vi "Final_Project_Intensity_Measurement.vi"() -> ()   [LabVIEW 2023]
doc: "This example shows how to get high accuracy DC voltage measurement."
uses:
  <instrlib>/Keithley DMM6500 DAQ6500 Series/Public/Data/Read (Single Point).vi
  <instrlib>/Keithley DMM6500 DAQ6500 Series/Keithley DMM6500 DAQ6500 Series.lvlib
panel:
  out "Intensity (W/m^2)":dbl
  out "Waveform Chart":dbl(graph)
  in  "stop":bool
  in  "Enable Average Filter (F: Disable)":bool
  in  "Input Impedance (0: 10Mohm)":i32(ring) items=["10Mohm", "Auto"]
  in  "Auto Zero (0: Enable)":u32(ring) items=["Enable", "Disable", "Once"]
  in  "Auto Range (T: Enable)":bool=TRUE
  in  "Average Filter Type (0: Repeat)":i32(ring) items=["Repeat", "Moving"]
  in  "Power Line Cycle (1)":dbl=10.0
  out "Voltage (V)":dbl
  in  "Average Count (10)":u32=10
  in  "Manual Range (0)":dbl=10.0
  in  "Channel List (\"101\")":string="101"
  in  "VISA resource name":refnum<visa-resource-name>
  # "(c) 2018-2022 National Instruments.  ALL RIGHTS RESERVED."
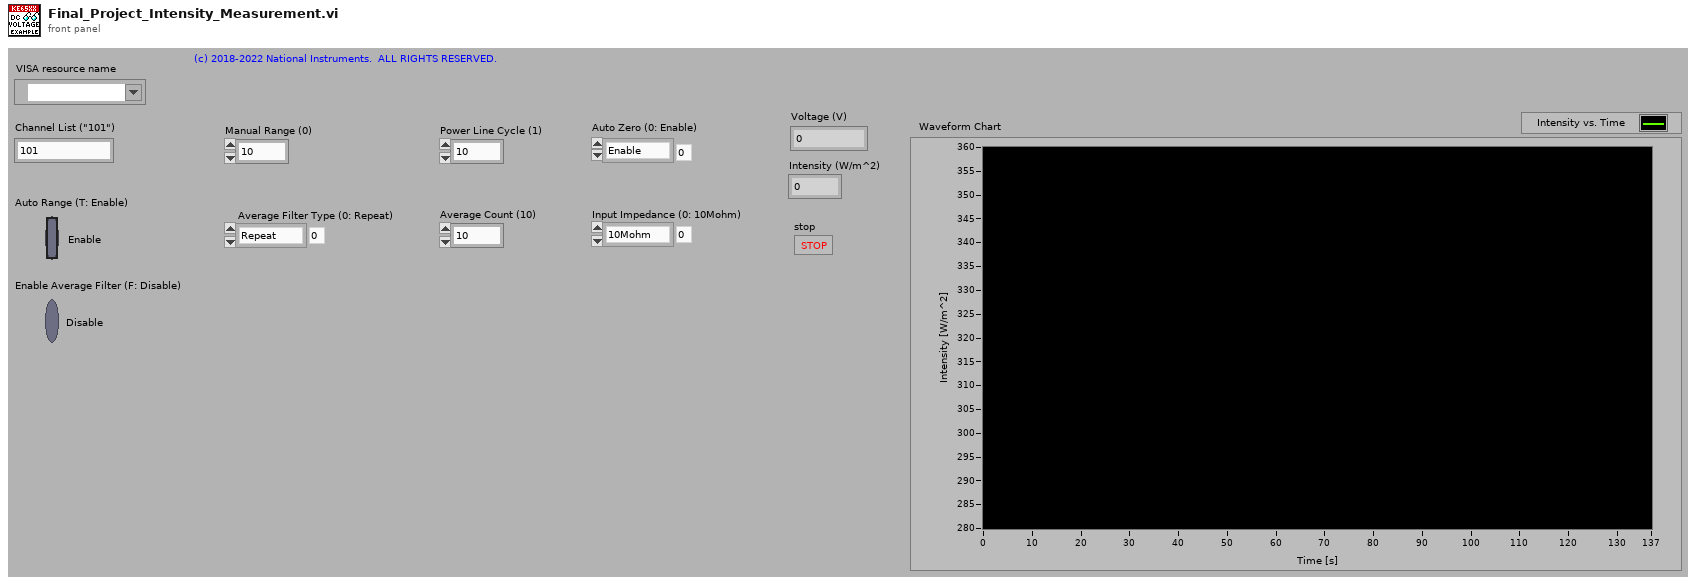
[diagram p1: front panel]
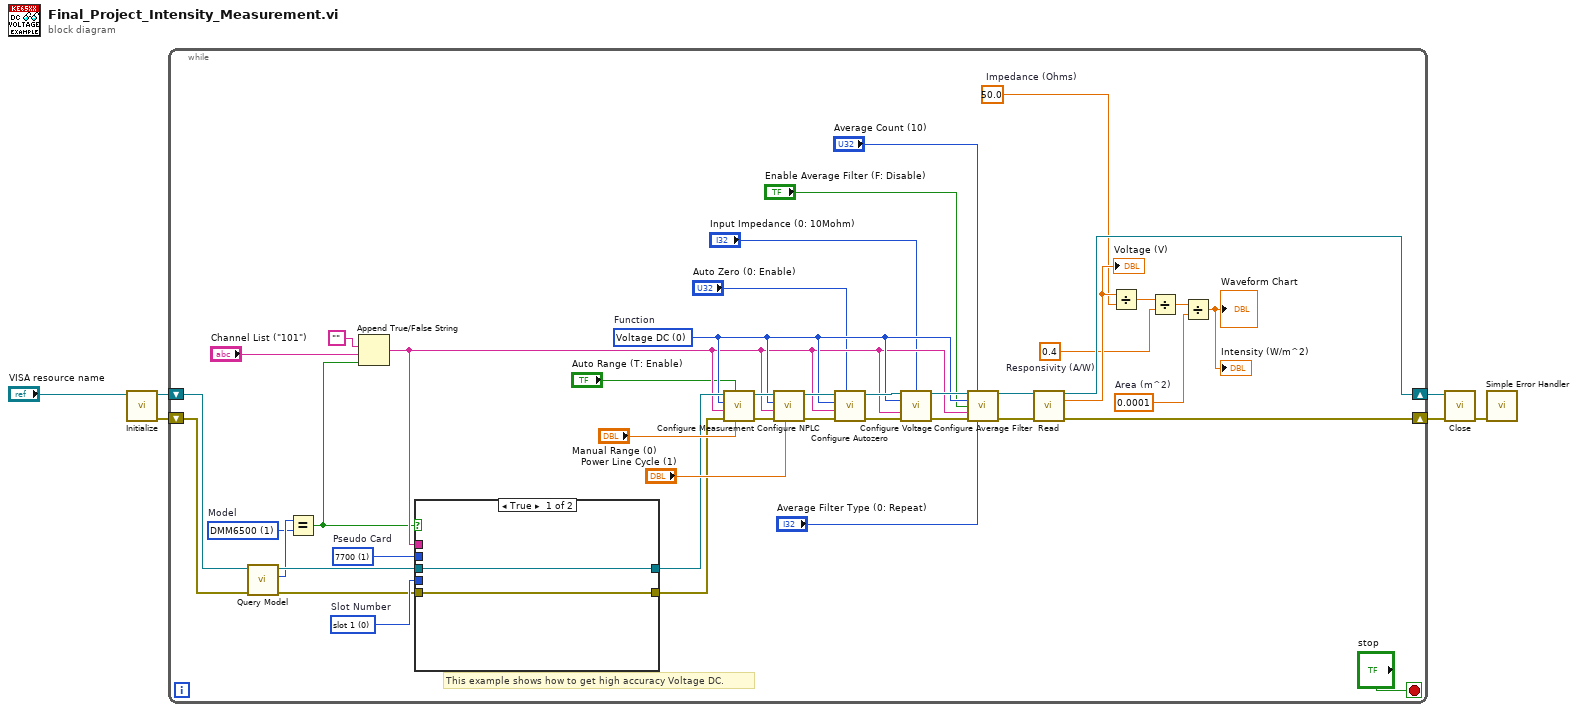
[diagram p0: block diagram]
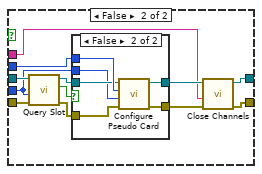
[diagram p2: hidden frame]
diagram:
  n1 = call <instrlib>:"Initialize.vi"("VISA resource name"="VISA resource name") -> ("error out"=w1:errorcluster, "VISA resource name out"=w2:refnum<visa-resource-name>)  [unwired: 9 in]
  n2 = while {
    shift-right: [w36] -> w3
    shift-left: w2 -> [w30]
    shift-right: [w37] -> w4
    shift-left: w1 -> [w28]
    stop <- "stop" stop-if-true
    w10 = 0.0001  # Area (m^2)
    w11 = 0.4  # Responsivity (A/W)
    w12 = 50.0  # Impedance (Ohms)
    w48 = 0 items=["slot 1", "slot 2"]  # Slot Number
    w49 = 1 items=["0", "7700", "7701", "7702", "7703", "7705", "7706", "7707", "7708", "7709", "7710", "7711", "7712"]  # Pseudo Card
    w24 = 0 items=[" Voltage DC", "Voltage AC", "Current DC", "Current AC", "Resistance", "4-wire Resistance", "Diode", "Capacitance", "Temperature", "Continuity", "Frequency", "Period", "Voltage Ratio", "Digitize Voltage", "Digitize Current"]  # Function
    w25 = 1 items=["", "DMM6500", "DAQ6510"]  # Model
    # "This example shows how to get high accuracy Voltage DC."
    n3 = call <instrlib>:"Query Model.vi"("error in (no error)"=w28, "VISA resource name"=w30) -> ("error out"=w27:errorcluster, "Model"=w26:i32, "VISA resource name out"=w29:refnum<visa-resource-name>)  [unwired: 7 in]
    n4 = Equal?(x=w26, y=w25) -> (x = y?=w20:bool)
    n5 = Append True/False String(1:w20, 2:"Channel List (\"101\")", 3:"") -> (0:w23:string)  [unwired: 1 in]
    n6 = case shown="True" w20 {
      tunnel: w49 -> [_ w63]
      tunnel: w48 -> [_ w53]
      tunnel: w29 -> [w51 w62]
      tunnel: w27 -> [w50 w55]
      tunnel: [w51 w60] -> w34
      tunnel: [w50 w58] -> w32
      tunnel: w23 -> [_ w57]
      frame True {
      }
      frame False {
        n7 = call <instrlib>:"Query Slot.vi"("error in (no error)"=w55, "Slot Number(0: slot 1)"=w53, "VISA resource name"=w62) -> ("error out"=w54:errorcluster, "Real Card In Slot"=w52:bool, "VISA resource name out"=w56:refnum<visa-resource-name>)  [unwired: 6 in]
        n8 = case shown="False" w52 {
          tunnel: w63 -> [_ w71]
          tunnel: [w65 w70] -> w61
          tunnel: [w64 w69] -> w59
          tunnel: w56 -> [w65 w68]
          tunnel: w54 -> [w64 w67]
          tunnel: w53 -> [_ w66]
          frame True {
          }
          frame False {
            n9 = call <instrlib>:"Configure Pseudo Card.vi"("error in (no error)"=w67, "Slot Number (0: slot1)"=w66, "Pseudo Card (0:No pseudocard)"=w71, "VISA resource name"=w68) -> ("error out"=w69:errorcluster, "VISA resource name out"=w70:refnum<visa-resource-name>)  [unwired: 6 in]
          }
        }
        n10 = call <instrlib>:"Close Channels.vi"("error in (no error)"=w59, "Channel List(\"\")"=w57, "VISA resource name"=w61) -> ("error out"=w58:errorcluster, "VISA resource name out"=w60:refnum<visa-resource-name>)  [unwired: 7 in]
      }
    }
    n11 = call <instrlib>:"Configure Measurement.vi"("Manual Range (1)"="Manual Range (0)", "Auto Range (T: Enable)"="Auto Range (T: Enable)", "error in (no error)"=w32, "Channel List(\"\")"=w23, "Function (0: Voltage DC)"=w24, "VISA resource name"=w34) -> ("error out"=w31:errorcluster, "VISA resource name out"=w33:refnum<visa-resource-name>)  [unwired: 4 in]
    n12 = call <instrlib>:"Configure NPLC.vi"("Power Line Cycle (1)"="Power Line Cycle (1)", "error in (no error)"=w31, "Channel List(\"\")"=w23, "Function (0: Voltage DC)"=w24, "VISA resource name"=w33) -> ("error out"=w45:errorcluster, "VISA resource name out"=w46:refnum<visa-resource-name>)  [unwired: 5 in]
    n13 = call <instrlib>:"Configure Autozero.vi"("Auto Zero (0: Enable)"="Auto Zero (0: Enable)", "error in (no error)"=w45, "Channel List(\"\")"=w23, "Function (0: Voltage DC)"=w24, "VISA resource name"=w46) -> ("error out"=w43:errorcluster, "VISA resource name out"=w44:refnum<visa-resource-name>)  [unwired: 5 in]
    n14 = call <instrlib>:"Configure Voltage.vi"("VISA resource name"=w44, "Input Impedance (0: 10Mohm)"="Input Impedance (0: 10Mohm)", "Function (0: Voltage DC)"=w24, "Channel List(\"\")"=w23, "error in (no error)"=w43) -> ("VISA resource name out"=w42:refnum<visa-resource-name>, "error out"=w41:errorcluster)  [unwired: 9 in]
    n15 = call <instrlib>:"Configure Average Filter.vi"("VISA resource name"=w42, "Count (10)"="Average Count (10)", "Function (0: Voltage DC)"=w24, "Enable Average Filter (F: Disable)"="Enable Average Filter (F: Disable)", "Channel List (\"\")"=w23, "error in (no error)"=w41, "Average Filter Type (0: Repeat)"="Average Filter Type (0: Repeat)") -> ("VISA resource name out"=w39:refnum<visa-resource-name>, "error out"=w38:errorcluster)  [unwired: 7 in]
    n16 = call-poly <instrlib>:"Read.vi"("VISA resource name"=w39, "error in (no error)"=w38) -> ("VISA resource name out"=w36:refnum<visa-resource-name>, "Measurement"=w13:dbl, "error out"=w37:errorcluster)  [unwired: 11 in]
    "Voltage (V)" <- w13
    n17 = Divide(x=w13, y=w12) -> (x/y=w8:dbl)
    n18 = Divide(x=w8, y=w11) -> (x/y=w9:dbl)
    n19 = Divide(x=w9, y=w10) -> (x/y=→"Waveform Chart" →"Intensity (W/m^2)":dbl)
  }
  n20 = call <instrlib>:"Close.vi"("error in (no error)"=w4, "VISA resource name"=w3) -> ("error out"=w6:errorcluster)  [unwired: 9 in]
  n21 = call <vilib>:"Simple Error Handler.vi"("error in (no error)"=w6) -> ()  [unwired: 4 in, 5 out]
